vi "Subset (DVR).vi"(8 "error in":errorcluster, 10 "Subset Slider (%)":cluster{dbl, dbl}(slide)={75.0, 25.0} scale=0.0..100.0 scale format="%#_6f", 11 "Data Value Reference in":refnum<data-value>) -> (0 "error out":errorcluster, 3 "Data Value Reference out":refnum<data-value>)   [LabVIEW 2016, in "Retrieve and Visualize.lvclass"]
uses:
  Retrieve and Visualize.lvclass
  <userlib>/LevyLab/XY Utilities/subVIs/Subset (multiple).vi
  <userlib>/LevyLab/XY Utilities/xy_utilities.lvlib
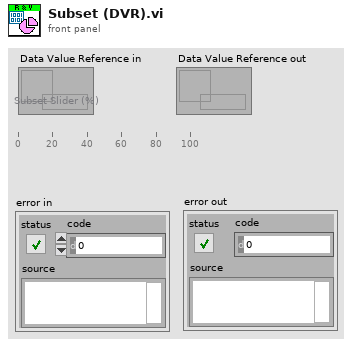
[diagram p1: front panel]
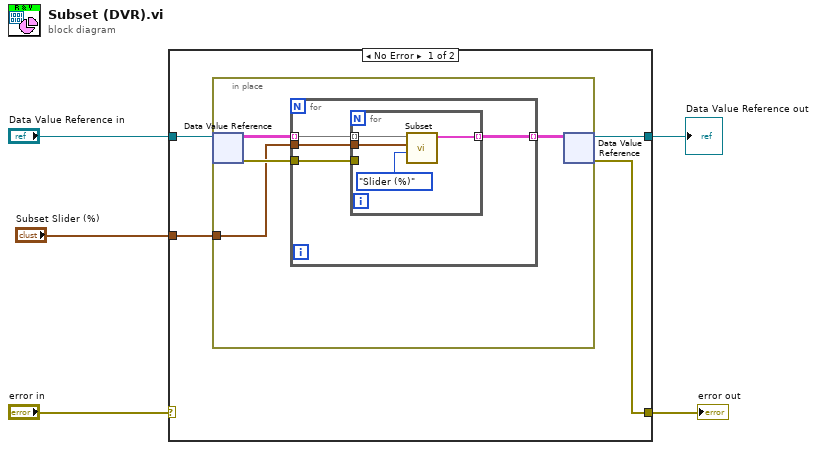
[diagram p0: block diagram]
diagram:
  n1 = case shown="No Error" "error in" {
    selector: "error in" -> [_ w23]
    tunnel: [w9 w22] -> w5
    tunnel: "Data Value Reference in" -> [w8 w22]
    tunnel: [w7 w23] -> w3
    tunnel: "Subset Slider (%)" -> [w6 _]
    frame No Error {
      n2 = in-place {
        in-place-border: w6 -> [w11]
        n3 = in-place-dvr #1(w8) -> (w13:cluster{dbl[], dbl[]}[][][], w12:errorcluster)
        n4 = for {
          tunnel: w13 -> [w17] mode=indexing
          tunnel: w12 -> [w16]
          tunnel: w11 -> [w15]
          tunnel: [w14] -> w10 mode=indexing
          n5 = for {
            tunnel: w17 -> [w19] mode=indexing
            tunnel: w16 -> [_]
            tunnel: w15 -> [w20]
            tunnel: [w18] -> w14 mode=indexing
            n6 = call-poly <userlib>:"Subset.vi"("Subset Method"=enum16{"Slider (%)", "X[] min and max"}."Slider (%)", "Subset Slider"=w20, "XY-data"=w19) -> ("Subset XY-data out"=w18:cluster{"X-array":dbl[], "Y-array":dbl[]}[])  [unwired: 7 in, 1 out]
          }
        }
        n7 = in-place-dvr #1(w10) -> (w9:refnum<data-value>, w7:errorcluster)
      }
    }
    frame Error {
    }
  }
  "Data Value Reference out" <- w5
  "error out" <- w3
